vi "HCSR04.vi"() -> ()   [LabVIEW 2015]
uses:
  <vilib>/MakerHub/LINX/Private/Device/Type Defs/Stimulus Pulse.ctl
  <vilib>/MakerHub/LINX/Public/Utilities/Open Serial.vi
  <vilib>/MakerHub/LINX/LMH-LINX.lvlib
  <vilib>/MakerHub/LINX/Private/Device/Device.lvlib
panel:
  out "SÜSPANSİYONU GEVŞET":bool
  out "SÜSPANSİYON SERBEST":bool
  out "SÜSPANSİYONU SERTLEŞTİR":bool
  in  "stop":bool
  out "MESAFE (cm)":u32
  in  "Serial Port":refnum<visa-resource-name>="N/A"
  in  "Echo":u8
  in  "Trigger":u8
  # "Designed by \nÖzkan Baykan"
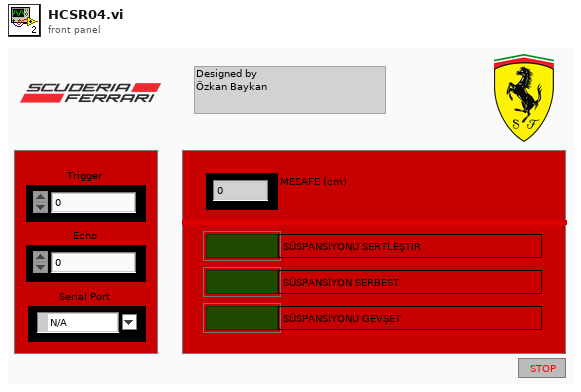
[diagram p1: front panel]
types:
  T1 = typedef "LMH-LINX.lvlib/LINX Ref.ctl" = cluster{"IO":T2, "Interface":T3, "LINX Device Config":T4}
  T2 = typedef "LMH-LINX.lvlib/Platform.ctl" = enum16{"Remote", "Local"}
  T3 = typedef "LMH-LINX.lvlib/Interface.ctl" = enum16{"Serial", "TCP"}
  T4 = typedef "LMH-LINX.lvlib/Device.lvlib/LINX Device Config.ctl" = cluster{"Interface":T3, "COM Port":refnum<visa-resource-name>, "TCP Configuration":T5, "Device Family":u8, "Device ID":u8, "Device Name":string, "TCP Ref":refnum<k5>, "Channels":T6}
  T5 = typedef "LMH-LINX.lvlib/Device.lvlib/TCP Config.ctl" = cluster{"IP Address":string, "Port":u16}
  T6 = typedef "LMH-LINX.lvlib/Channels.ctl" = cluster{"DI":u8[], "DO":u8[], "AI":u8[], "AO":u8[], "PWM":u8[], "QE":u8[], "UART":u8[], "I2C 2":u8[], "SPI":u8[], "CAN":u8[], "Servo":u8[], "AI Ref (V)":dbl, "AI Resolution (Bits)":u8, "AO Ref (V)":dbl, "AO Resolution (Bits)":u8}
  T7 = typedef "LMH-LINX.lvlib/Device.lvlib/Stimulus Pulse.ctl" = enum16{"None", "Active Low", "Active High"}
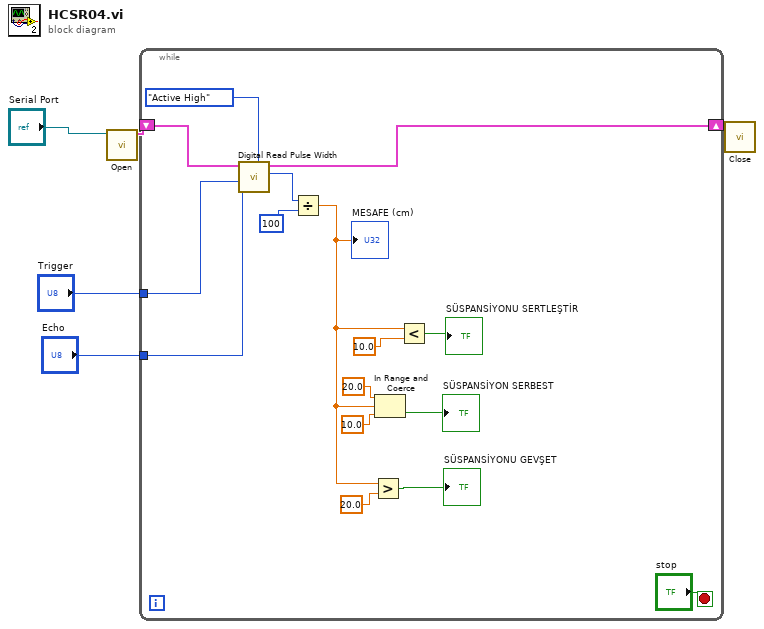
[diagram p0: block diagram]
diagram:
  n1 = call-poly <vilib>:"Open.vi"("Serial Port"="Serial Port") -> ("LINX Resource"=w2:T1)  [unwired: 8 in, 2 out]
  n2 = while {
    tunnel: "Trigger" -> [w21]
    tunnel: "Echo" -> [w20]
    shift-right: [w19] -> w3
    shift-left: w2 -> [w18]
    stop <- "stop" stop-if-true
    n3 = call <vilib>:"Digital Read Pulse Width.vi"("Stimulus Pulse (Active High)"=Stimulus_Pulse."Active High", "DO Channel"=w21, "DI Channel"=w20, "LINX Resource"=w18) -> ("Pulse Width (uS)"=w15:u32, "LINX Resource"=w19:T1)  [unwired: 5 in, 1 out]
    n4 = Divide(x=w15, y=100) -> (x/y=w7:dbl)
    "MESAFE (cm)" <- w7
    n5 = Greater?(x=w7, y=20.0) -> (0:→"SÜSPANSİYONU GEVŞET":bool)
    n6 = In Range and Coerce(upper limit=20.0, x=w7, lower limit=10.0) -> (In Range?=→"SÜSPANSİYON SERBEST":bool)  [unwired: 1 out]
    n7 = Less?(x=w7, y=10.0) -> (x < y?=→"SÜSPANSİYONU SERTLEŞTİR":bool)
  }
  n8 = call <vilib>:"Close.vi"("LINX Resource"=w3) -> ()  [unwired: 10 in, 1 out]
